vi "Configure Route Single.vi"(0 "VISA resource name":refnum<visa-resource-name>, 1 "Operation (0: Open All)":u16(ring) items=["Open All", "Open", "Close"], 2 "Channel (1)":i32=1, 5 "error in (no error)":errorcluster) -> (14 "VISA resource name out":refnum<visa-resource-name>, 19 "error out":errorcluster)   [LabVIEW 2018, in "Keithley 2000.lvlib"]
doc: "This VI controls the switch functionality of an internal or external scanner card. It can be used to open or close one or more channels.\n\nNote:\nThis is a polymorphic VI. You can wire a single channel number or an array of channel numbers to configure multiple channels at once."
uses:
  <instrlib>/Keithley 2000/Keithley 2000.lvlib
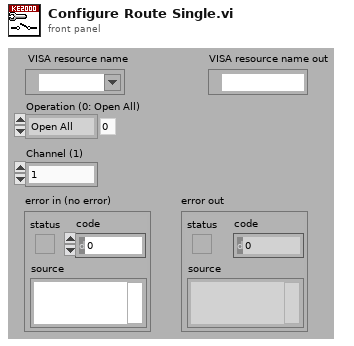
[diagram p1: front panel]
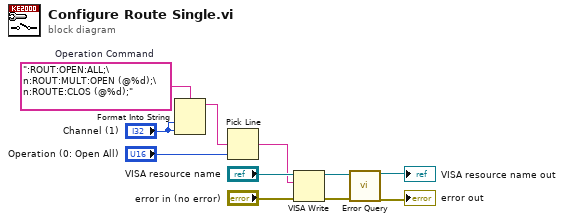
[diagram p0: block diagram]
diagram:
  w9 = ":ROUT:OPEN:ALL;\n:ROUT:MULT:OPEN (@%d);\n:ROUTE:CLOS (@%d);"  # Operation Command
  n1 = Format Into String(format string=w9, "Channel (1)", "Channel (1)") -> (resulting string=w7:string)  [unwired: 2 in, 1 out]
  n2 = Pick Line(multi-line string=w7, line index="Operation (0: Open All)") -> (output string=w5:string)  [unwired: 1 in]
  n3 = VISA Write(VISA resource name="VISA resource name", write buffer=w5, error in (no error)="error in (no error)") -> (VISA resource name out=w4:refnum<visa-resource-name>, error out=w1:errorcluster)  [unwired: 1 out]
  n4 = call <instrlib>:"Error Query.vi"("VISA resource name"=w4, "error in (no error)"=w1) -> ("VISA resource name out"=→"VISA resource name out":refnum<visa-resource-name>, "error out"=→"error out":errorcluster)  [unwired: 14 in, 2 out]
